vi "List Log Files.vi"(8 "error in (no error)":errorcluster, 10 "extension":string="csv", 11 "rootFolder":path) -> (0 "error out":errorcluster, 2 "count":i32, 3 "filePaths":path[](array[path]))   [LabVIEW 2026, in "Tests.lvlib"]
doc: "Test readback helper for file-mechanics tests. Recursively lists log files under a root folder matching the given extension, returned sorted by path, so tests can assert how many files were written and where (including calendar sub-folders created when calendarFolderTree is enabled). Call only after Shutdown has flushed and closed the files, the appender holds the current file open until CloseSink. Pure read; does not modify the tree."
uses:
  Tests.lvlib
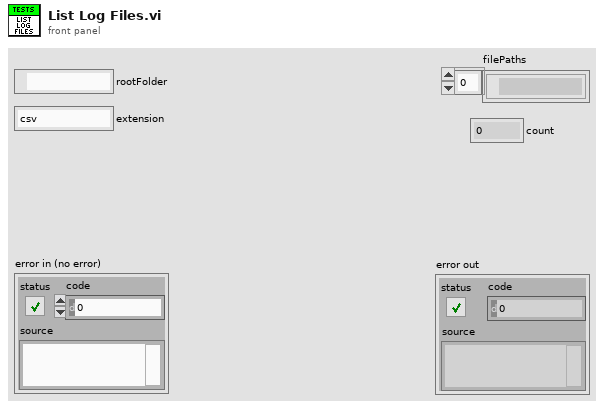
[diagram p1: front panel]
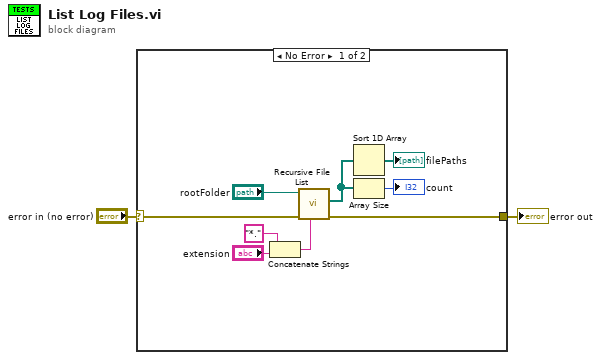
[diagram p0: block diagram]
diagram:
  n1 = case shown="No Error" "error in (no error)" {
    selector: "error in (no error)" -> [w5 w12]
    tunnel: [w11 w12] -> w2
    frame No Error {
      n2 = Concatenate Strings("*." ("pattern"), "extension") -> (w7:string)
      n3 = call <vilib>:"Recursive File List.vi"("pattern"=w7, "error in (no error)"=w5, "Folder Path"="rootFolder") -> ("error out"=w11:errorcluster, "All Files in Dir"=w4:path[])  [unwired: 4 in, 3 out]
      n4 = Sort 1D Array(array=w4) -> (sorted array=→"filePaths":path[])
      n5 = Array Size(array=w4) -> (size(s)=→"count":i32)
    }
    frame Error {
    }
  }
  "error out" <- w2
